vi "OpenDBL.vi"(2 "Action":u16(ring) items=["Get Image", "Load and Read File"]) -> (4 "Image":sgl[](array[numeric]), 8 "Physical Length (Z, Y, X, t)":sgl[](array[numeric]), 15 "Dimensions (Z, Y, X, t)":i32[](array[numeric]))   [LabVIEW 2014]
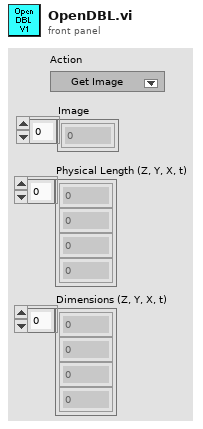
[diagram p1: front panel]
types:
  T1 = enum16{"big-endian, network order", "native, host order", "little-endian"}
  T2 = enum16{"open", "replace", "create", "open or create", "replace or create", "replace or create with confirmation"}
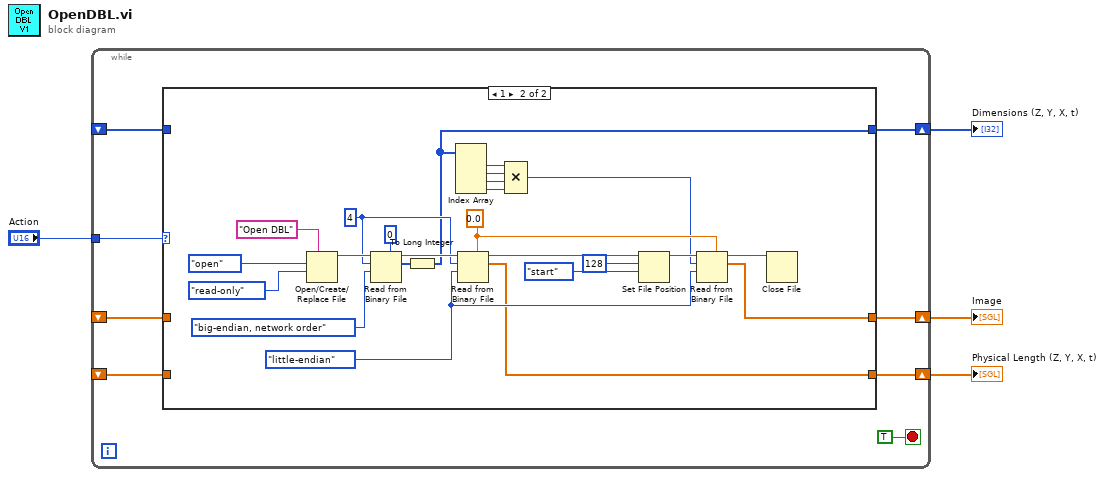
[diagram p0: block diagram]
diagram:
  n1 = while {
    shift-right: [w10] -> w1
    shift-left: _ -> [w7]
    shift-right: [w8] -> w2
    shift-left: _ -> [w6]
    shift-right: [w9] -> w3
    shift-left: _ -> [w5]
    tunnel: "Action" -> [w11]
    stop <- TRUE stop-if-true
    n2 = case shown="1" w11 {
      tunnel: [w13 w23] -> w9
      tunnel: [w15 w17] -> w10
      tunnel: [w14 w21] -> w8
      tunnel: w7 -> [w15 _]
      tunnel: w6 -> [w14 _]
      tunnel: w5 -> [w13 _]
      frame 0, Default {
      }
      frame 1 {
        w29 = sgl 0.0
        w27 = T1."little-endian" ("byte order (0:big-endian, network order)")
        w30 = 4 ("count (1)")
        n3 = Open/Create/Replace File(prompt="Open DBL", operation (0:open)=T2."open", access (0:read/write)=enum16{"read/write", "read-only", "write-only"}."read-only") -> (refnum out=w36:refnum<file>)  [unwired: 3 in, 2 out]
        n4 = Read from Binary File(5:u16 0, 9:T1."big-endian, network order" ("byte order (0:big-endian, network order)"), 10:w30, 11:w36) -> (2:w22:u16[], 3:w33:refnum<file>)  [unwired: 2 in, 2 out]
        n5 = To Long Integer(number=w22) -> (32bit integer=w17:i32[])
        n6 = Index Array(array=w17) -> (element #1=w18:i32, element #2=w19:i32, element #3=w25:i32, element #4=w24:i32)  [unwired: 4 in]
        n7 = Read from Binary File(5:w29, 9:w27, 10:w30, 11:w33) -> (2:w23:sgl[], 3:w32:refnum<file>)  [unwired: 2 in, 2 out]
        n8 = Compound Arithmetic op=MULTIPLY(w18, w19, w25, w24) -> (w16:i32)
        n9 = Set File Position(offset (in bytes) (0)=i64 128, refnum=w32, from (0:start)=enum16{"start", "end", "current"}."start") -> (refnum out=w20:refnum<file>)  [unwired: 1 in, 1 out]
        n10 = Read from Binary File(5:w29, 9:w27, 10:w16, 11:w20) -> (2:w21:sgl[], 3:w26:refnum<file>)  [unwired: 2 in, 2 out]
        n11 = Close File(refnum=w26) -> ()  [unwired: 1 in, 2 out]
      }
    }
  }
  "Dimensions (Z, Y, X, t)" <- w1
  "Physical Length (Z, Y, X, t)" <- w3
  "Image" <- w2
